vi "User Utilities Button.vi"() -> (3 "MenuOutput":string)   [LabVIEW 2023]
uses:
  Controls/DisplayQCommand.ctl
  Controls/DisplayMessage.ctl
panel:
  in  "User Utils":bool
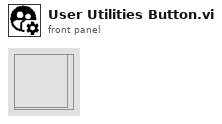
[diagram p1: front panel]
types:
  T1 = typedef "DisplayMessage.ctl" = enum16{"No Message - Ignore", "Display Message", "Set Tab", "Set Status", "Add Error Message", "Clear Error History", "Generate Error", "Set Idling Display", "Set Running Display", "Set Subpanel Output", "Stop"}
  T2 = typedef "DisplayQCommand.ctl" = enum16{"No Command - Error", "Initialise", "Get Q Reference", "Add Item to Bottom", "Add Item to Top", "Flush Q", "Dequeue", "Peek Next Element", "Close"}
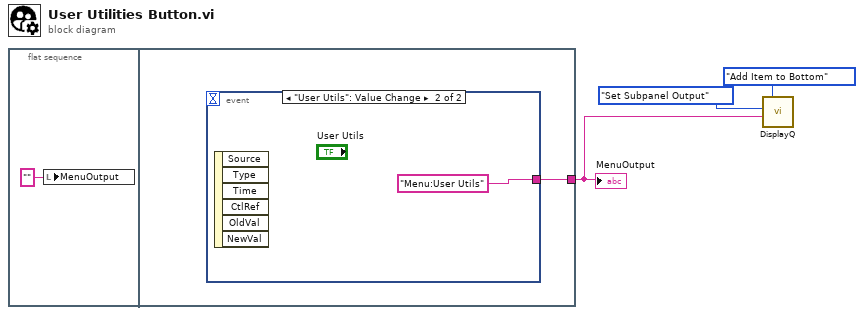
[diagram p0: block diagram]
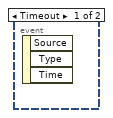
[diagram p2: hidden frame]
diagram:
  n1 = flat-sequence {
    tunnel: [w5] -> w2
    frame #0 {
      n2 = local write "MenuOutput"("" ("MenuOutput")) -> ()
    }
    frame #1 {
      n3 = event shown="[1] \"User Utils\": Value Change" {
        selector: _ -> [_ _]
        dyn-events: _ -> [_ _]
        timeout: _ -> [_ _]
        tunnel: [_ "Menu:User Utils"] -> w5
        event Timeout {
          n4 = event-data() -> ()  [unwired: 1 in, 3 out]
        }
        event "User Utils": Value Change {
          n5 = event-data() -> ()  [unwired: 1 in, 6 out]
        }
      }
    }
  }
  n6 = call "DisplayQ.vi"("command"=DisplayQCommand."Add Item to Bottom", "DataIn"=w2, "DisplayMessage"=DisplayMessage."Set Subpanel Output") -> ()  [unwired: 2 in, 4 out]
  "MenuOutput" <- w2
